vi "List Packages.vi"(7 "LabVIEW Web Service Request":refnum<class "Web Request.lvclass">) -> ()   [LabVIEW 2016]
uses:
  <vilib>/wsapi/Web Request.lvclass
  Libraries/WSsupport/Search Filters.ctl
  Libraries/Packages/Repo_class/Repo.lvclass/Repo.ctl
  Libraries/Packages/Repo_class/Read Packages.vi
  <vilib>/addons/JSON API/JSON Scalar/JSON Scalar.lvclass
  C:/Program Files (x86)/National Instruments/LabVIEW 2016/vi.lib/addons/JSON API/JSON Value/JSON Value.lvclass
  <vilib>/addons/JSON API/JSON Array/JSON Array.lvclass
  <vilib>/addons/JSON API/JSON Object/JSON Object.lvclass
  Libraries/WSsupport/GV_Repos.vi
  Libraries/Packages/Package_class/Package.lvclass
  Libraries/WSsupport/WSsupport.lvlib
  <vilib>/addons/JSON API/JSON Value/JSON Value.lvclass
  Libraries/ServerErrors/ServerErrors.lvlib
  Libraries/Packages/Repo_class/Repo.lvclass
panel:
  # "Use the Web Service Request input terminal to call the VIs on the Web Services palette. Do not remove it from the connector pane unless you don't need access to the palette."
  # "Each additional control wired to the connector pane will be available as an input in the URL. To include an indicator in terminal-mode output (the default setting), it must also be wired to the connector pane."
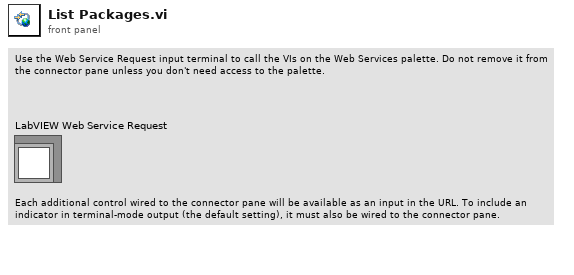
[diagram p1: front panel]
types:
  T1 = typedef "WSsupport.lvlib/Search Filters.ctl" = cluster{"RepoTypes":string[], "RepoNames":string[]}
  T2 = cluster{"PageNumber":i32, "SearchCriteria":string, "Filters":T1}
  T3 = typedef "ServerErrors.lvlib/Error Message--cluster.ctl" = cluster{"HTTP Code":i32, "JSON Response":cluster{"error":string, "reason":string}}
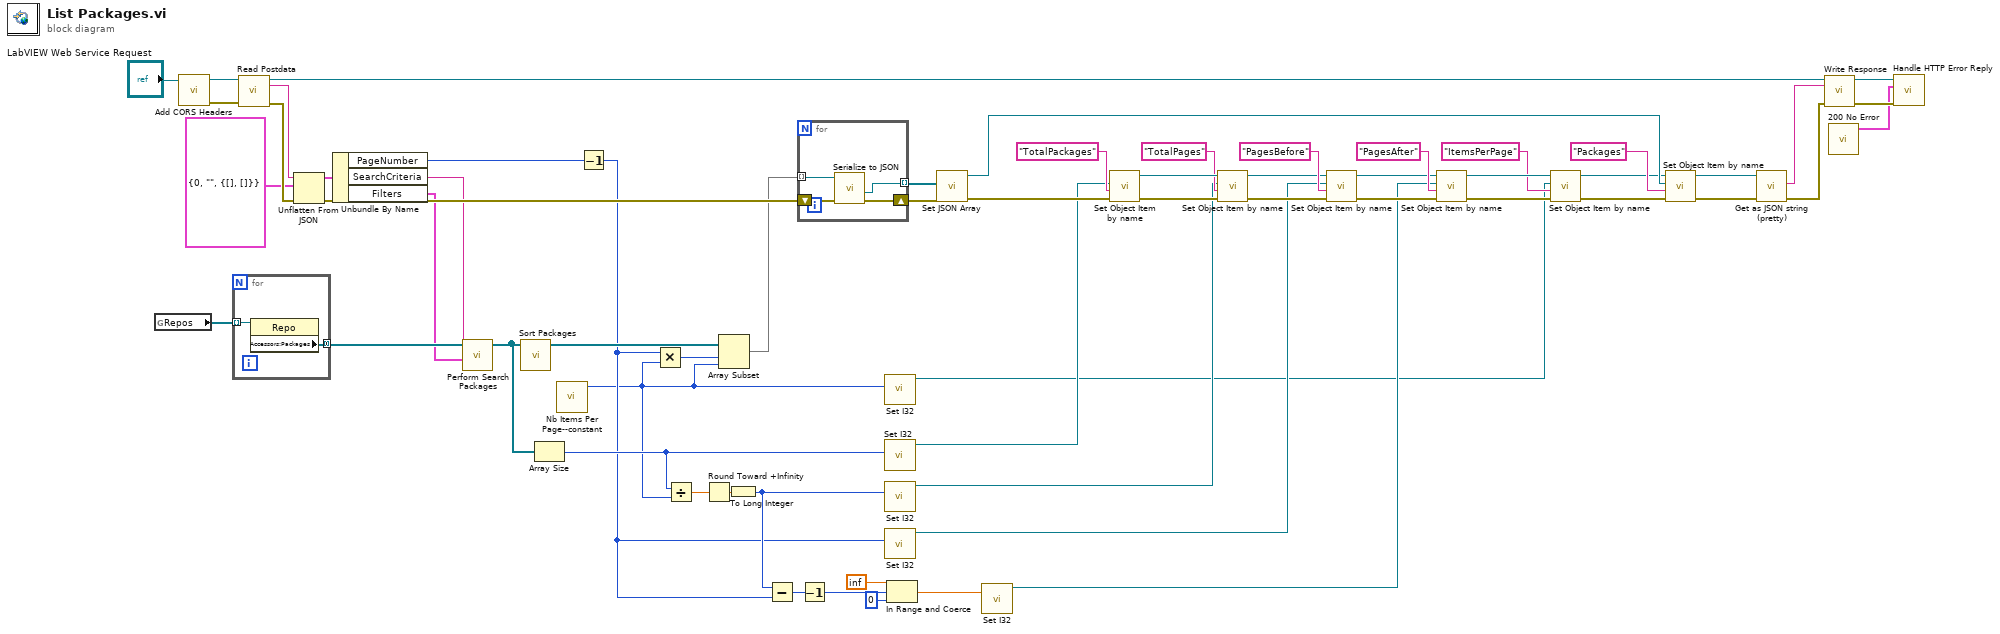
[diagram p0: block diagram]
diagram:
  n1 = global read "GV_Repos.vi" "Repos"() -> (w45:refnum<class "Repo.lvclass">[])
  n2 = call "Add CORS Headers.vi"("LabVIEW Web Service Request"="LabVIEW Web Service Request") -> ("error out"=w60:errorcluster, "LabVIEW Web Service Request out"=w50:refnum<class "Web Request.lvclass">)  [unwired: 9 in]
  n3 = for {
    tunnel: w45 -> [w63] mode=indexing
    tunnel: [w62] -> w33 mode=concatenating
    n4 = property class="Repo"(reference=w63) -> ("Accessors:Packages"=w62:refnum<class "Package.lvclass">[])  [unwired: 1 in, 2 out]
  }
  n5 = call <vilib>:"Read Postdata.vi"("LabVIEW Web Service Request"=w50, "error in (no error)"=w60) -> ("LabVIEW Web Service Request out"=w49:refnum<class "Web Request.lvclass">, "postdata"=w17:string, "error out"=w51:errorcluster)  [unwired: 11 in]
  n6 = Unflatten From JSON(JSON string=w17, type and defaults=T2 {"PageNumber"=0, "SearchCriteria"="", "Filters"={"RepoTypes"=[], "RepoNames"=[]}}, error in (no error)=w51) -> (value=w46:T2, error out=w48:errorcluster)  [unwired: 4 in]
  n7 = Unbundle By Name(w46) -> ("PageNumber"=w43:i32, "SearchCriteria"=w9:string, "Filters"=w1:T1)
  n8 = call "Perform Search Packages.vi"("Filters"=w1, "SearchCriteria"=w9, "All Packages"=w33) -> ("Found Packages"=w2:refnum<class "Package.lvclass">[])  [unwired: 8 in]
  n9 = call "Sort Packages.vi"("Packages"=w2) -> ("Sorted Packages"=w44:refnum<class "Package.lvclass">[])  [unwired: 10 in]
  n10 = Array Size(array=w2) -> (size(s)=w27:i32)
  n11 = call "Nb Items Per Page--constant.vi"() -> ("Nb Items Per Page"=w5:i32)  [unwired: 11 in]
  n12 = Decrement(x=w43) -> (x-1=w21:i32)
  n13 = Multiply(x=w21, y=w5) -> (x*y=w42:i32)
  n14 = Divide(x=w27, y=w5) -> (x/y=w26:dbl)
  n15 = Round Toward +Infinity(x=w26) -> (ceil(x): smallest int >= x=w25:dbl)
  n16 = Array Subset(array=w44, index=w42, length=w5) -> (w41:refnum<class "Package.lvclass">[])
  n17 = To Long Integer(number=w25) -> (32bit integer=w22:i32)
  n18 = Subtract(x=w22, y=w21) -> (x-y=w20:i32)
  n19 = for {
    tunnel: w41 -> [w65] mode=indexing
    shift-right: [w66] -> w59
    shift-left: w48 -> [w67]
    tunnel: [w64] -> w58 mode=indexing
    n20 = call-dynamic "Serialize to JSON.vi"("error in (no error)"=w67, "Package in"=w65) -> ("error out"=w66:errorcluster, "JSON Value"=w64:refnum<class "JSON Value.lvclass">)  [unwired: 6 in, 2 out]
  }
  n21 = Decrement(x=w20) -> (x-1=w19:i32)
  n22 = call <vilib>:"Set I32.vi"("Numeric"=w5) -> ("JSON Scalar out"=w3:refnum<class "JSON Scalar.lvclass">)  [unwired: 9 in, 1 out]
  n23 = call <vilib>:"Set I32.vi"("Numeric"=w27) -> ("JSON Scalar out"=w32:refnum<class "JSON Scalar.lvclass">)  [unwired: 9 in, 1 out]
  n24 = call <vilib>:"Set I32.vi"("Numeric"=w22) -> ("JSON Scalar out"=w24:refnum<class "JSON Scalar.lvclass">)  [unwired: 9 in, 1 out]
  n25 = call <vilib>:"Set I32.vi"("Numeric"=w21) -> ("JSON Scalar out"=w23:refnum<class "JSON Scalar.lvclass">)  [unwired: 9 in, 1 out]
  n26 = In Range and Coerce(upper limit=inf, x=w19, lower limit=0) -> (coerced(x)=w16:dbl)  [unwired: 1 out]
  n27 = call <vilib>:"Set JSON Array.vi"("error in (no error)"=w59, "Array"=w58) -> ("error out"=w57:errorcluster, "JSON Array out"=w10:refnum<class "JSON Array.lvclass">)  [unwired: 8 in]
  n28 = call <vilib>:"Set I32.vi"("Numeric"=w16) -> ("JSON Scalar out"=w18:refnum<class "JSON Scalar.lvclass">)  [unwired: 9 in, 1 out]
  n29 = call <vilib>:"Set Object Item by name.vi"("error in (no error)"=w57, "name"="TotalPackages", "Value"=w32) -> ("error out"=w40:errorcluster, "JSON Object out"=w30:refnum<class "JSON Object.lvclass">)  [unwired: 6 in, 1 out]
  n30 = call <vilib>:"Set Object Item by name.vi"("error in (no error)"=w40, "name"="TotalPages", "Value"=w24, "JSON Object in"=w30) -> ("error out"=w31:errorcluster, "JSON Object out"=w29:refnum<class "JSON Object.lvclass">)  [unwired: 5 in, 1 out]
  n31 = call <vilib>:"Set Object Item by name.vi"("error in (no error)"=w31, "name"="PagesBefore", "Value"=w23, "JSON Object in"=w29) -> ("error out"=w38:errorcluster, "JSON Object out"=w34:refnum<class "JSON Object.lvclass">)  [unwired: 5 in, 1 out]
  n32 = call <vilib>:"Set Object Item by name.vi"("error in (no error)"=w38, "name"="PagesAfter", "Value"=w18, "JSON Object in"=w34) -> ("error out"=w36:errorcluster, "JSON Object out"=w7:refnum<class "JSON Object.lvclass">)  [unwired: 5 in, 1 out]
  n33 = call <vilib>:"Set Object Item by name.vi"("error in (no error)"=w36, "name"="ItemsPerPage", "Value"=w3, "JSON Object in"=w7) -> ("error out"=w8:errorcluster, "JSON Object out"=w6:refnum<class "JSON Object.lvclass">)  [unwired: 5 in, 1 out]
  n34 = call <vilib>:"Set Object Item by name.vi"("error in (no error)"=w8, "name"="Packages", "Value"=w10, "JSON Object in"=w6) -> ("error out"=w13:errorcluster, "JSON Object out"=w12:refnum<class "JSON Object.lvclass">)  [unwired: 5 in, 1 out]
  n35 = call <vilib>:"Get as JSON string (pretty).vi"("error in (no error)"=w13, "JSON Value in"=w12) -> ("error out"=w52:errorcluster, "<JSON>"=w56:string)  [unwired: 8 in]
  n36 = call <vilib>:"Write Response.vi"("LabVIEW Web Service Request"=w49, "response string"=w56, "error in (no error)"=w52) -> ("LabVIEW Web Service Request out"=w55:refnum<class "Web Request.lvclass">, "error out"=w54:errorcluster)  [unwired: 11 in]
  n37 = call "200 No Error.vi"() -> ("no error"=w53:T3)  [unwired: 11 in]
  n38 = call "Handle HTTP Error Reply.vi"("error in (no error)"=w54, "HTTP Status Code"=w53, "Web Request in"=w55) -> ()  [unwired: 8 in, 1 out]
